vi "Configure Shutter State.vi"(8 "error in (no error)":errorcluster, 9 "Enable Shutter State (F:OFF)":bool, 10 "Platform Slot Number (10)":i16=10 min=-1 max=255, 11 "VISA resource name":refnum<visa-resource-name>) -> (0 "error out":errorcluster, 3 "VISA resource name out":refnum<visa-resource-name>)   [LabVIEW 2018, in "LTB-1.lvlib" / "3150.lvlib"]
doc: "Configures the state of the instrument's shutter (open or closed). The shutter is used to let light through the input or block it."
uses:
  3150.lvlib
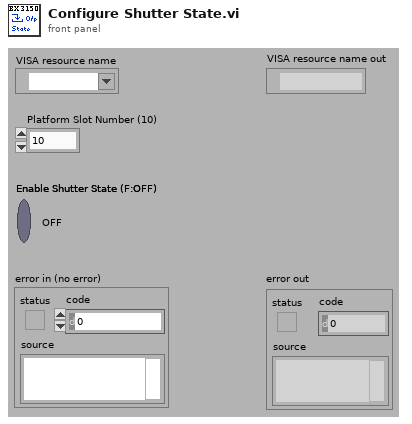
[diagram p1: front panel]
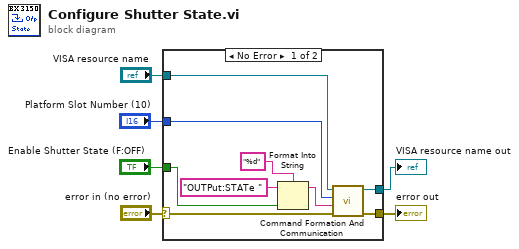
[diagram p0: block diagram]
diagram:
  n1 = case shown="No Error" "error in (no error)" {
    selector: "error in (no error)" -> [w14 w16]
    tunnel: "VISA resource name" -> [w15 w17]
    tunnel: [w13 w17] -> w4
    tunnel: [w12 w16] -> w3
    tunnel: "Enable Shutter State (F:OFF)" -> [w10 _]
    tunnel: "Platform Slot Number (10)" -> [w7 _]
    frame No Error {
      n2 = Format Into String(format string="%d", initial string="OUTPut:STATe " ("Command"), w10) -> (resulting string=w8:string)  [unwired: 1 in, 1 out]
      n3 = call "Command Formation And Communication.vi"("error in (no error)"=w14, "Command"=w8, "Platform Slot Number"=w7, "VISA resource name"=w15) -> ("error out"=w12:errorcluster, "VISA resource name out"=w13:refnum<visa-resource-name>)  [unwired: 1 in, 5 out]
    }
    frame Error {
    }
  }
  "VISA resource name out" <- w4
  "error out" <- w3
